vi "To String.vi"(8 "error in (no error)":errorcluster, 11 "SnailNum in":refnum<class "SnailNum.lvclass">) -> (0 "error out":errorcluster, 2 "String":string, 3 "SnailNum out":refnum<class "SnailNum.lvclass">)   [LabVIEW 2020, in "SnailNum.lvclass"]
uses:
  SnailNum.lvclass
  SnailNum.lvclass/SnailNum.ctl
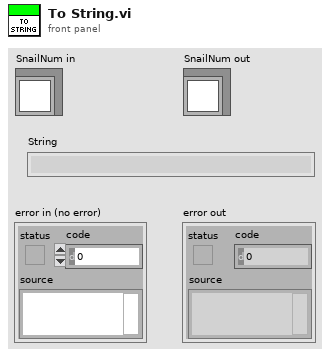
[diagram p1: front panel]
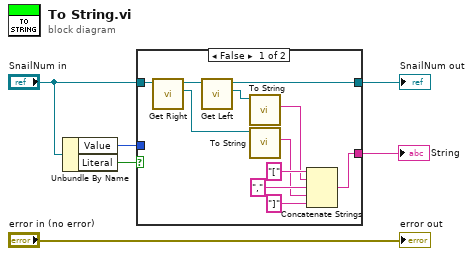
[diagram p0: block diagram]
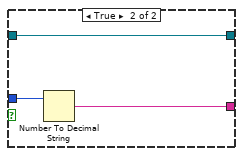
[diagram p2: hidden frame]
diagram:
  n1 = Unbundle By Name("SnailNum in") -> ("Value"=w4:i64, "Literal"=w5:bool)
  n2 = case shown="False" w5 {
    tunnel: w4 -> [_ w20]
    tunnel: [w7 w19] -> w3
    tunnel: "SnailNum in" -> [w14 w18]
    tunnel: [w12 w18] -> w1
    frame False {
      n3 = call "Get Right.vi"("SnailNum in"=w14) -> ("Right"=w10:refnum<class "SnailNum.lvclass">, "SnailNum out"=w13:refnum<class "SnailNum.lvclass">)  [unwired: 8 in, 1 out]
      n4 = call "Get Left.vi"("SnailNum in"=w13) -> ("Left"=w11:refnum<class "SnailNum.lvclass">, "SnailNum out"=w12:refnum<class "SnailNum.lvclass">)  [unwired: 8 in, 1 out]
      n5 = call "To String.vi"("SnailNum in"=w11) -> ("String"=w9:string)  [unwired: 8 in, 2 out]
      n6 = call "To String.vi"("SnailNum in"=w10) -> ("String"=w8:string)  [unwired: 8 in, 2 out]
      n7 = Concatenate Strings("[" ("string"), w9, "," ("string"), w8, "]" ("string")) -> (w7:string)
    }
    frame True {
      n8 = Number To Decimal String(number=w20) -> (decimal integer string=w19:string)  [unwired: 1 in]
    }
  }
  "SnailNum out" <- w1
  "String" <- w3
  "error out" <- "error in (no error)"
